vi "ReadConfiguration.vi"(5 "回放路径：":path) -> (0 "增益":i64=227, 1 "曝光时间(us)":i64, 2 "帧率/FPS":dbl, 3 "帧间隔/us":i64=200000 min=100000 max=500000 step=1, 4 "PacketSize":u32=1500, 6 "总帧数":dbl)   [LabVIEW 2012]
uses:
  <vilib>/Utility/xml.llb/Read From XML File(array).vi
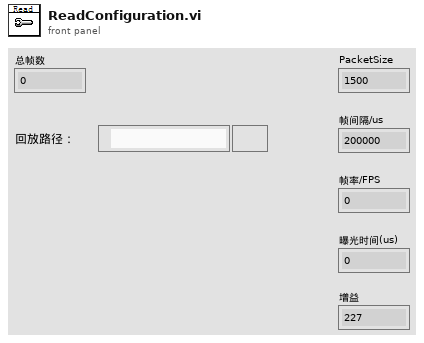
[diagram p1: front panel]
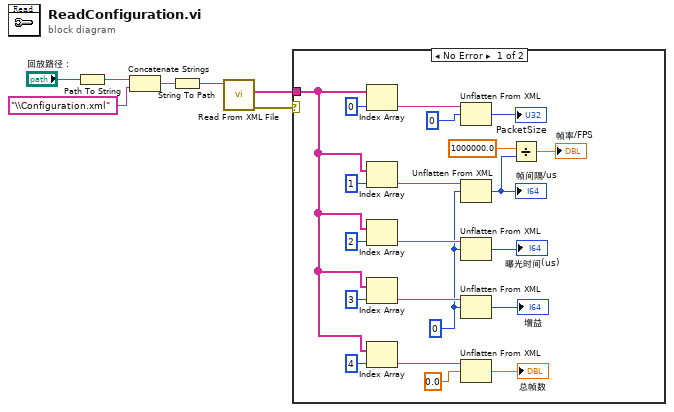
[diagram p0: block diagram]
diagram:
  n1 = Path To String(path="回放路径：") -> (string=w6:string)
  n2 = Concatenate Strings(w6, "\\Configuration.xml" ("字符串")) -> (w4:string)
  n3 = String To Path(string=w4) -> (path=w3:path)
  n4 = call-poly <vilib>:"Read From XML File.vi"("XML File Path"=w3) -> ("error out"=w2:errorcluster, "XML Elements"=w1:string[])  [unwired: 8 in, 1 out]
  n5 = case shown="No Error" w2 {
    tunnel: w1 -> [w12 _]
    frame No Error {
      w10 = i64 0
      n6 = Index Array(array=w12, index=0 ("索引")) -> (element=w24:string)
      n7 = Index Array(array=w12, index=1 ("索引")) -> (element=w22:string)
      n8 = Index Array(array=w12, index=2 ("索引")) -> (element=w21:string)
      n9 = Index Array(array=w12, index=3 ("索引")) -> (element=w20:string)
      n10 = Index Array(array=w12, index=4 ("索引")) -> (element=w11:string)
      n11 = Unflatten From XML(xml string=w24, type=u32 0) -> (value=→"PacketSize":u32)  [unwired: 1 in, 1 out]
      n12 = Unflatten From XML(xml string=w22, type=w10) -> (value=w18:i64)  [unwired: 1 in, 1 out]
      "帧间隔/us" <- w18
      n13 = Unflatten From XML(xml string=w21, type=w10) -> (value=→"曝光时间(us)":i64)  [unwired: 1 in, 1 out]
      n14 = Unflatten From XML(xml string=w20, type=w10) -> (value=→"增益":i64)  [unwired: 1 in, 1 out]
      n15 = Unflatten From XML(xml string=w11, type=0.0) -> (value=→"总帧数":dbl)  [unwired: 1 in, 1 out]
      n16 = Divide(x=1000000.0, y=w18) -> (x/y=→"帧率/FPS":dbl)
    }
    frame Error {
    }
  }
